vi "ExositionCalc.vi"(11 "A(8)axis":dbl[](array[numeric])) -> (3 "A(8)axis":dbl)   [LabVIEW 2019]
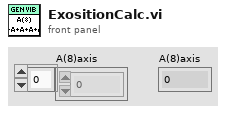
[diagram p1: front panel]
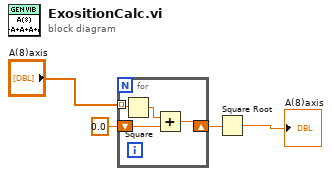
[diagram p0: block diagram]
diagram:
  n1 = for {
    tunnel: "A(8)axis" -> [w8] mode=indexing
    shift-right: [w6] -> w3
    shift-left: 0.0 -> [w5]
    n2 = Square(x=w8) -> (x^2=w7:dbl)
    n3 = Add(x=w7, y=w5) -> (x+y=w6:dbl)
  }
  n4 = Square Root(x=w3) -> (sqrt(x)=→"A(8)axis":dbl)
